vi "XML_ValidateCompleteness.vi"(8 "Tag":string="TransformerObj", 11 "XML":T1) -> (2 "valid?":bool, 3 "XML out":string)   [LabVIEW 2017]
doc: "Returns TRUE when XML contains both the opening and the closing tag of the element named Tag, which detects a truncated document."
uses:
  _XML--String.ctl
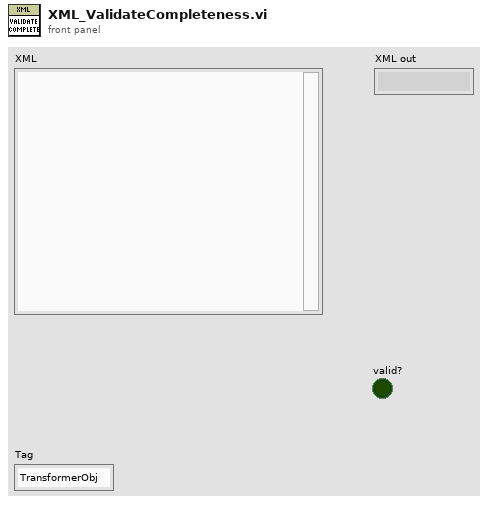
[diagram p1: front panel]
types:
  T1 = typedef "_XML--String.ctl" = string
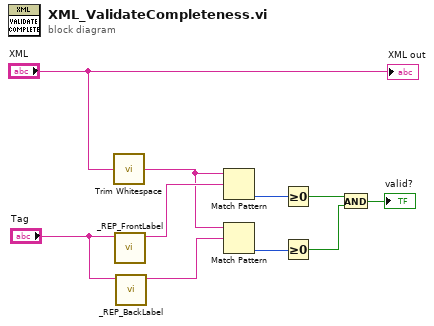
[diagram p0: block diagram]
diagram:
  n1 = call <vilib>:"Trim Whitespace.vi"("string"="XML") -> ("trimmed string"=w8:string)  [unwired: 1 in]
  n2 = call "_REP_FrontLabel.vi"("label"="Tag") -> ("String"=w10:string)  [unwired: 10 in]
  n3 = call "_REP_BackLabel.vi"("label"="Tag") -> ("String"=w7:string)  [unwired: 10 in]
  n4 = Match Pattern(string=w8, regular expression=w10) -> (offset past match=w6:i32)  [unwired: 1 in, 3 out]
  n5 = Match Pattern(string=w8, regular expression=w7) -> (offset past match=w5:i32)  [unwired: 1 in, 3 out]
  n6 = Greater Or Equal To 0?(x=w6) -> (x >= 0?=w3:bool)
  n7 = Greater Or Equal To 0?(x=w5) -> (x >= 0?=w4:bool)
  n8 = And(x=w3, y=w4) -> (x .and. y?=→"valid?":bool)
  "XML out" <- "XML"
